vi "Test Report UTF8 Compatibility.vi"(8 "error in (no error)":errorcluster) -> (0 "error out":errorcluster, 3 "UTF8 Compatible":bool)   [LabVIEW 2020]
uses:
  classes/Test Suite/Define Test Suite (SimpleText Report).vi
  classes/Test Suite/Test Suite.lvclass
panel:
  out "utf-8 text":string
  out "Test Report File Contents":string
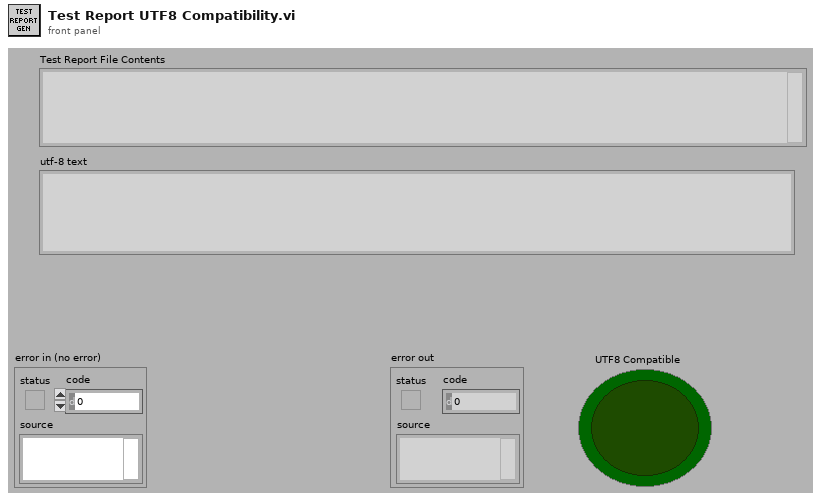
[diagram p1: front panel]
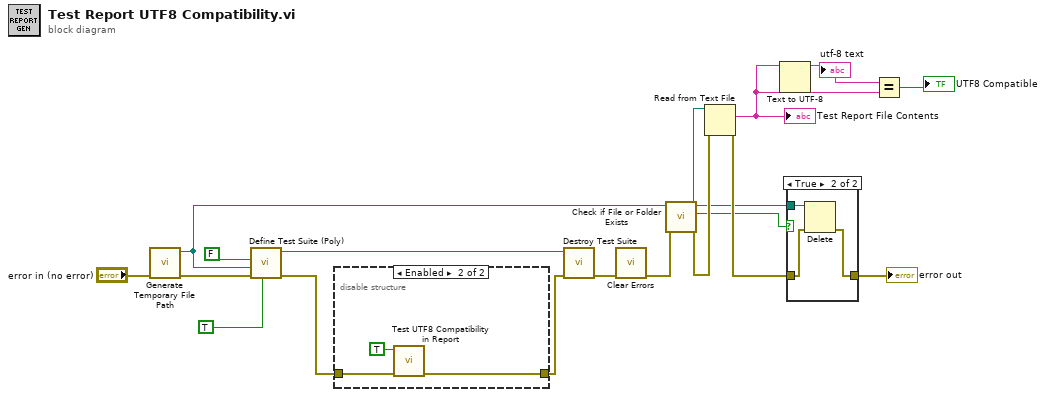
[diagram p0: block diagram]
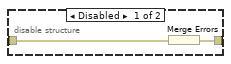
[diagram p2: hidden frame]
diagram:
  n1 = call <vilib>:"Generate Temporary File Path.vi"("error in (no error)"="error in (no error)") -> ("error out"=w11:errorcluster, "Unique Temporary File Path"=w10:path)  [unwired: 9 in]
  n2 = call-poly "Define Test Suite (Poly).vi"("Verbose (F)"=TRUE, "error in (no error)"=w11, "Report Path"=w10, "Interactive"=FALSE) -> ("error out"=w8:errorcluster, "Test Suite"=w12:refnum<class "Test Suite.lvclass">)  [unwired: 5 in, 1 out]
  n3 = disable-structure shown="Enabled" {
    disable-tunnel: [w20 w22] -> w9
    disable-tunnel: w8 -> [w19 w23]
    frame Disabled {
      n4 = Merge Errors(w19) -> (w20:errorcluster)
    }
    frame Enabled {
      n5 = call "Test UTF8 Compatibility in Report.vi"("error in (no error)"=w23, "Force FAIL?"=TRUE) -> ("error out"=w22:errorcluster)  [unwired: 9 in]
    }
  }
  n6 = call-dynamic "Destroy Test Suite.vi"("error in (no error)"=w9, "Test Suite in"=w12) -> ("error out"=w6:errorcluster)  [unwired: 8 in, 1 out]
  n7 = call <vilib>:"Clear Errors.vi"("error in (no error)"=w6) -> ("error out"=w5:errorcluster)  [unwired: 5 in, 1 out]
  n8 = call <vilib>:"Check if File or Folder Exists.vi"("error in (no error)"=w5, "path"=w10) -> ("error out"=w16:errorcluster, "file or folder exists?"=w2:bool, "dup path"=w14:path)  [unwired: 7 in]
  n9 = Read from Text File(file (use dialog)=w14, error in=w16) -> (text=w3:string, error out=w15:errorcluster)  [unwired: 2 in, 2 out]
  "Test Report File Contents" <- w3
  n10 = Text to UTF-8(11:w3) -> (3:w4:string)  [unwired: 2 in, 1 out]
  "utf-8 text" <- w4
  n11 = case shown="True" w2 {
    tunnel: w14 -> [_ w27]
    tunnel: w15 -> [w24 w26]
    tunnel: [w24 w25] -> w17
    frame False {
    }
    frame True {
      n12 = Delete(path (use dialog)=w27, error in=w26) -> (error out=w25:errorcluster)  [unwired: 3 in, 2 out]
    }
  }
  "error out" <- w17
  n13 = Equal?(x=w4, y=w3) -> (x = y?=→"UTF8 Compatible":bool)
